vi "Get Popup.vi"(8 "error in (no error)":errorcluster caption="错误输入（无错误）", 10 "Point":T1, 11 "Popup 输入":refnum<class "Popup.lvclass"> caption="DNL_LabVIEW Object in") -> (0 "error out":errorcluster caption="错误输出", 3 "Popup 输出":refnum<class "Popup.lvclass"> caption="DNL_LabVIEW Object out")   [LabVIEW 2017, in "Popup.lvclass"]
uses:
  Popup.lvclass
  <vilib>/Utility/miscctls.llb/LVPositionTypeDef.ctl
  Popup.lvclass/Popup.ctl
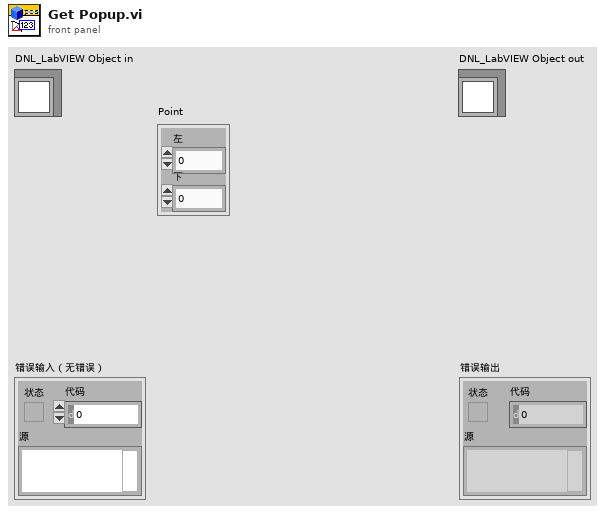
[diagram p1: front panel]
types:
  T1 = typedef "LVPositionTypeDef.ctl" = cluster{"Left":i32, "Top":i32}
  T2 = typedef "LVRowAndColumnTypeDef.ctl" = cluster{"Row":i32, "Column":i32}
  T3 = typedef "LVBoundsTypeDef.ctl" = cluster{"Width":u32, "Height":u32}
  T4 = typedef "LVFontTypeDef.ctl" = cluster{"Font Name":string, "Size":u16, "Bold":bool, "Italic":bool, "Underline":bool, "Strikeout":bool, "Color":u32}
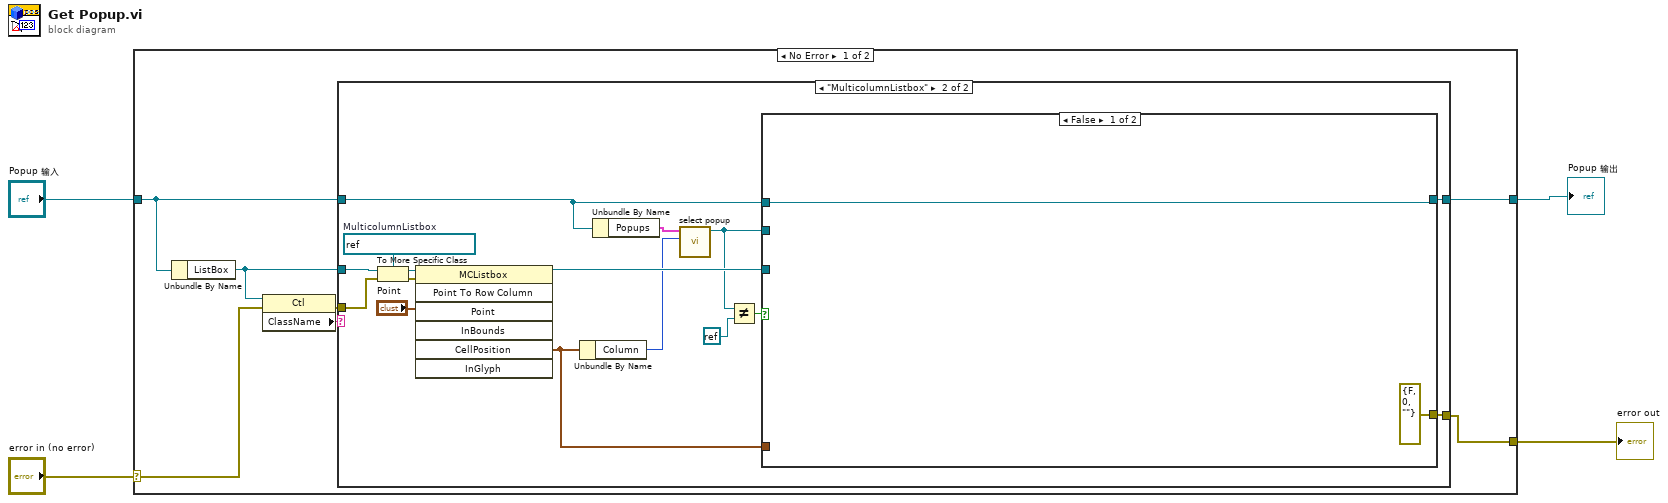
[diagram p0: block diagram]
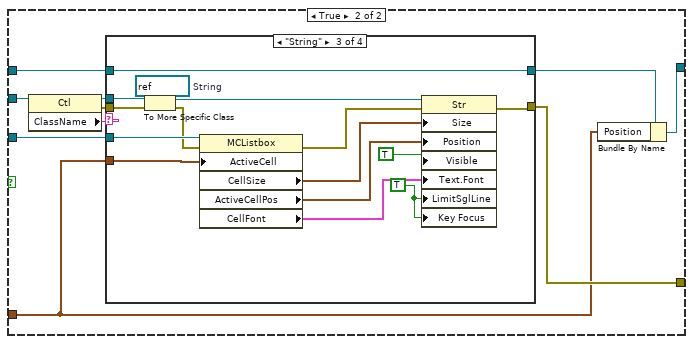
[diagram p3: hidden frame]
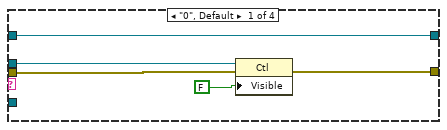
[diagram p4: hidden frame]
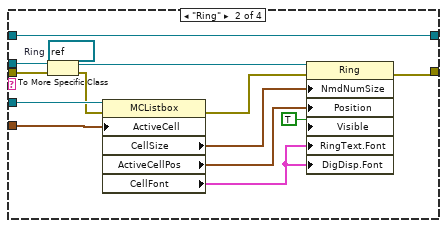
[diagram p5: hidden frame]
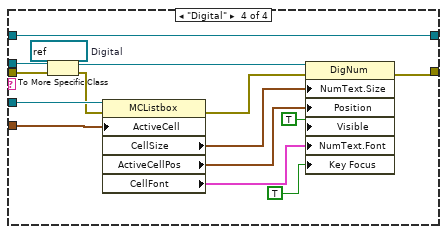
[diagram p6: hidden frame]
diagram:
  n1 = case shown="No Error" "error in (no error)" {
    selector: "error in (no error)" -> [w8 w92]
    tunnel: [w5 w92] -> w3
    tunnel: [w10 w91] -> w1
    tunnel: "Popup 输入" -> [w11 w91]
    frame No Error {
      n2 = Unbundle By Name(w11) -> ("ListBox"=w9:refnum<vi>)
      n3 = property class="Ctl"(reference=w9, error in=w8) -> (error out=w6:errorcluster, "ClassName"=w7:string)  [unwired: 1 out]
      n4 = case shown="\"MulticolumnListbox\"" w7 {
        tunnel: w11 -> [w13 w25]
        tunnel: [w12 w23] -> w5
        tunnel: [w13 w22] -> w10
        tunnel: w9 -> [_ w20]
        tunnel: w6 -> [w12 w19]
        frame "假", Default {
        }
        frame "MulticolumnListbox" {
          w29 = refnum<vi> refnum  # MulticolumnListbox
          n5 = To More Specific Class(target class=w29, reference=w20, error in=w19) -> (specific class reference=w28:refnum<vi>, error out=w27:errorcluster)
          n6 = invoke class="MCListbox" method="Point To Row Column"(reference=w28, error in=w27, "Point"="Point") -> (reference out=w24:refnum<vi>, "CellPosition"=w21:T2)  [unwired: 4 in, 5 out]
          n7 = Unbundle By Name(w21) -> ("Column"=w17:i32)
          n8 = Unbundle By Name(w25) -> ("Popups"=w18:cluster{"Referens":refnum<vi>, "Column":i32}[])
          n9 = call "select popup.vi"("Column"=w17, "Popups"=w18) -> ("Ring输出"=w15:refnum<vi>)  [unwired: 9 in]
          n10 = Not Equal?(x=w15, y=refnum<k0> refnum) -> (x != y?=w16:bool)
          n11 = case shown="False" w16 {
            tunnel: w25 -> [w31 w41]
            tunnel: w24 -> [_ w40]
            tunnel: [errorcluster {"status"=FALSE, "code"=0, "source"=""} ("error out") w39] -> w23
            tunnel: [w31 w37] -> w22
            tunnel: w21 -> [_ w36]
            tunnel: w15 -> [_ w35]
            frame False {
            }
            frame True {
              n12 = property class="Ctl"(reference=w35) -> (reference out=w32:refnum<vi>, error out=w34:errorcluster, "ClassName"=w33:string)  [unwired: 1 in]
              n13 = case shown="\"String\"" w33 {
                tunnel: w41 -> [w42 w56 w71 w86]
                tunnel: w32 -> [w46 w50 w65 w80]
                tunnel: w34 -> [w45 w51 w66 w81]
                tunnel: w40 -> [_ w60 w75 w90]
                tunnel: [w43 w57 w72 w87] -> w39
                tunnel: [w42 w56 w71 w86] -> w38
                tunnel: w36 -> [_ w59 w74 w89]
                frame "0", Default {
                  n14 = property class="Ctl"(reference=w46, error in=w45, "Visible"=FALSE) -> (error out=w43:errorcluster)  [unwired: 1 out]
                }
                frame "Ring" {
                  w49 = refnum<vi> refnum  # Ring
                  n15 = To More Specific Class(target class=w49, reference=w50, error in=w51) -> (specific class reference=w48:refnum<vi>, error out=w47:errorcluster)
                  n16 = property class="MCListbox"(reference=w60, error in=w47, "ActiveCell"=w59) -> (error out=w58:errorcluster, "CellSize"=w55:T3, "ActiveCellPos"=w54:T1, "CellFont"=w52:T4)  [unwired: 1 out]
                  n17 = property class="Ring"(reference=w48, error in=w58, "NmdNumSize"=w55, "Position"=w54, "Visible"=TRUE, "RingText.Font"=w52, "DigDisp.Font"=w52) -> (error out=w57:errorcluster)  [unwired: 1 out]
                }
                frame "String" {
                  w61 = TRUE
                  w64 = refnum<vi> refnum  # String
                  n18 = To More Specific Class(target class=w64, reference=w65, error in=w66) -> (specific class reference=w63:refnum<vi>, error out=w62:errorcluster)
                  n19 = property class="MCListbox"(reference=w75, error in=w62, "ActiveCell"=w74) -> (error out=w73:errorcluster, "CellSize"=w70:T3, "ActiveCellPos"=w69:T1, "CellFont"=w67:T4)  [unwired: 1 out]
                  n20 = property class="Str"(reference=w63, error in=w73, "Size"=w70, "Position"=w69, "Visible"=TRUE, "Text.Font"=w67, "LimitSglLine"=w61, "Key Focus"=w61) -> (error out=w72:errorcluster)  [unwired: 1 out]
                }
                frame "Digital" {
                  w79 = refnum<vi> refnum  # Digital
                  n21 = To More Specific Class(target class=w79, reference=w80, error in=w81) -> (specific class reference=w78:refnum<vi>, error out=w77:errorcluster)
                  n22 = property class="MCListbox"(reference=w90, error in=w77, "ActiveCell"=w89) -> (error out=w88:errorcluster, "CellSize"=w85:T3, "ActiveCellPos"=w84:T1, "CellFont"=w82:T4)  [unwired: 1 out]
                  n23 = property class="DigNum"(reference=w78, error in=w88, "NumText.Size"=w85, "Position"=w84, "Visible"=TRUE, "NumText.Font"=w82, "Key Focus"=TRUE) -> (error out=w87:errorcluster)  [unwired: 1 out]
                }
              }
              n24 = Bundle By Name(cluster=w38, "Position"=w36) -> (w37:refnum<class "Popup.lvclass">)
            }
          }
        }
      }
    }
    frame Error {
    }
  }
  "error out" <- w3
  "Popup 输出" <- w1
